vi "列表框-滚动条更新(LV8.6).vi"() -> ()   [LabVIEW 2018]
panel:
  in  "停止":bool
  in  "列表框":i32(listbox)
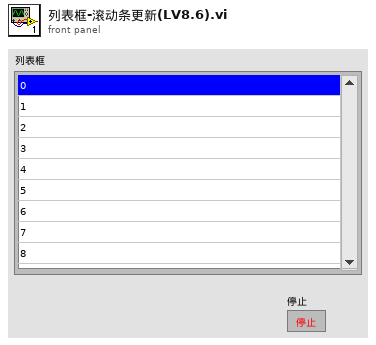
[diagram p1: front panel]
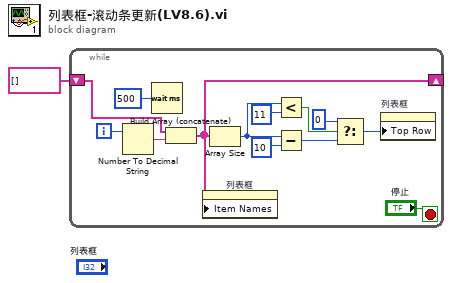
[diagram p0: block diagram]
diagram:
  n1 = while {
    shift-right: [w12] -> _
    shift-left: string[] [] -> [w11]
    i -> [w9]
    stop <- "停止" stop-if-true
    n2 = Number To Decimal String(number=w9) -> (decimal integer string=w10:string)  [unwired: 1 in]
    n3 = Wait (ms)(milliseconds to wait=u32 500 ("等待时间（毫秒）")) -> ()  [unwired: 1 out]
    n4 = Build Array (concatenate)(w11, w10) -> (w12:string[])
    n5 = property on="列表框" class="LstBox (严格)"("Item Names"=w12) -> ()  [unwired: 2 in, 2 out]
    n6 = Array Size(array=w12) -> (size(s)=w4:i32)
    n7 = Less?(x=w4, y=11) -> (x < y?=w6:bool)
    n8 = Subtract(x=w4, y=10) -> (x-y=w5:i32)
    n9 = Select(t=0, s=w6, f=w5) -> (s? t:f=w3:i32)
    n10 = property on="列表框" class="LstBox (严格)"("Top Row"=w3) -> ()  [unwired: 2 in, 2 out]
  }
